vi "PH_Stepmotor_BaseClass.Convert Steps.vi"(0 "Postion (steps)":i32, 1 "Calibration Factor":dbl) -> (2 "Scaled Position":dbl)   [LabVIEW 2014, in "PH_Stepmotor_BaseClass.lvlib"]
uses:
  PH_Stepmotor_BaseClass.lvlib
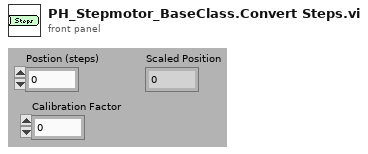
[diagram p1: front panel]
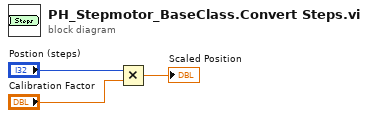
[diagram p0: block diagram]
diagram:
  n1 = Multiply(x="Postion (steps)", y="Calibration Factor") -> (x*y=→"Scaled Position":dbl)
